vi "Concatenate result strings.vi"(7 "Location":enum16{"Start", "End"}(ring), 8 "Message":string, 9 "Description":string, 10 "Status":T1, 11 "Input String":string) -> (3 "Output String":string)   [LabVIEW 2020, in "Method Result.lvclass"]
uses:
  Method Result.lvclass
  Assertion Result/Public/TypeDefs/Status.ctl
  Assertion Result/Assertion Result.lvclass
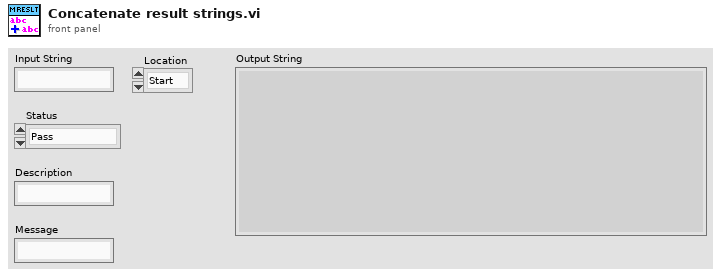
[diagram p1: front panel]
types:
  T1 = typedef "Assertion Result.lvclass/Status.ctl" = enum16{"Pass", "Fail", "Error", "Skipped", "Setup Error", "Broken", "Teardown Error"}
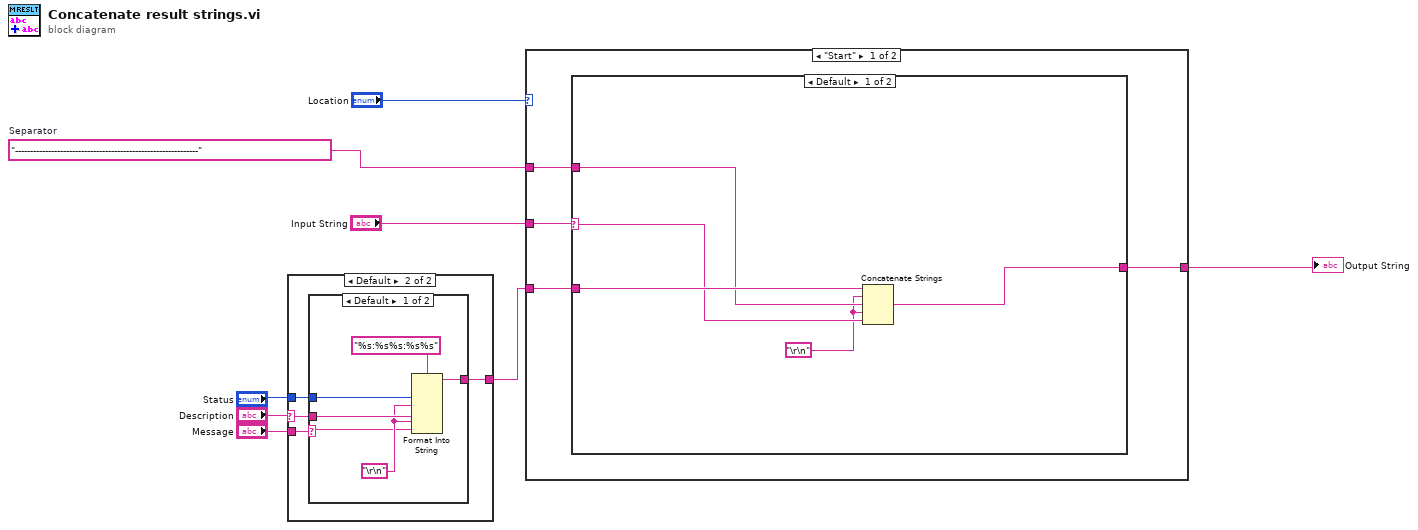
[diagram p0: block diagram]
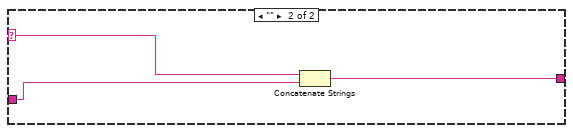
[diagram p2: hidden frame]
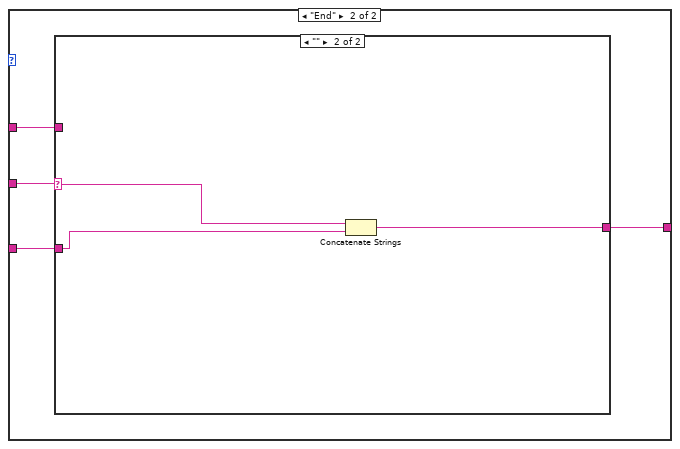
[diagram p3: hidden frame]
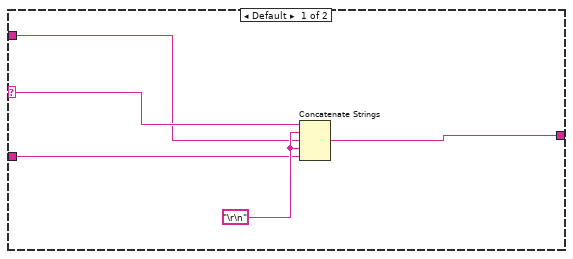
[diagram p4: hidden frame]
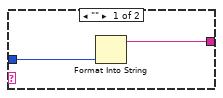
[diagram p5: hidden frame]
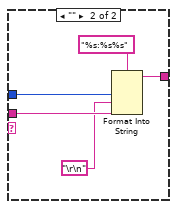
[diagram p6: hidden frame]
diagram:
  w7 = "-------------------------------------------------------------"  # Separator
  n1 = case shown="Default" "Description" {
    selector: "Description" -> [_ w13]
    tunnel: "Status" -> [w10 w14]
    tunnel: "Message" -> [_ w12]
    tunnel: [w9 w11] -> w2
    frame "" {
      n2 = Format Into String(w10) -> (resulting string=w9:string)  [unwired: 3 in, 1 out]
    }
    frame Default {
      n3 = case shown="Default" w12 {
        selector: w12 -> [w17 _]
        tunnel: w14 -> [w20 w24]
        tunnel: w13 -> [w19 w23]
        tunnel: [w16 w21] -> w11
        frame Default {
          w18 = "\r\n"
          n4 = Format Into String(format string="%s:%s%s:%s%s", w20, w18, w19, w18, w17) -> (resulting string=w16:string)  [unwired: 2 in, 1 out]
        }
        frame "" {
          n5 = Format Into String(format string="%s:%s%s", w24, "\r\n", w23) -> (resulting string=w21:string)  [unwired: 2 in, 1 out]
        }
      }
    }
  }
  n6 = case shown="\"Start\"" "Location" {
    tunnel: w7 -> [w27 w39]
    tunnel: "Input String" -> [w29 w41]
    tunnel: w2 -> [w28 w40]
    tunnel: [w26 w38] -> w1
    frame "Start" {
      n7 = case shown="Default" w29 {
        selector: w29 -> [w31 w35]
        tunnel: w28 -> [w34 w37]
        tunnel: w27 -> [w33 _]
        tunnel: [w32 w36] -> w26
        frame Default {
          w30 = "\r\n"
          n8 = Concatenate Strings(w34, w30, w33, w30, w31) -> (w32:string)
        }
        frame "" {
          n9 = Concatenate Strings(w35, w37) -> (w36:string)
        }
      }
    }
    frame "End" {
      n10 = case shown="\"\"" w41 {
        selector: w41 -> [w45 w47]
        tunnel: w40 -> [w43 w49]
        tunnel: w39 -> [w42 _]
        tunnel: [w46 w48] -> w38
        frame Default {
          w44 = "\r\n"
          n11 = Concatenate Strings(w45, w44, w42, w44, w43) -> (w46:string)
        }
        frame "" {
          n12 = Concatenate Strings(w47, w49) -> (w48:string)
        }
      }
    }
  }
  "Output String" <- w1
